vi "err_log.vi"(5 "error IO 2":errorcluster, 6 "time stamp":timestamp) -> (1 "err_table":string[](array[string]))   [LabVIEW 2010]
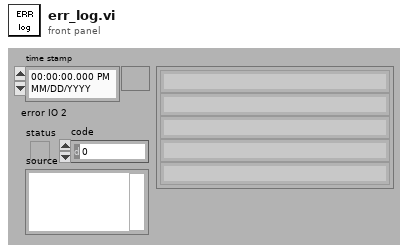
[diagram p1: front panel]
types:
  T1 = enum16{"open", "replace", "create", "open or create", "replace or create", "replace or create with confirmation"}
  T2 = cluster{"status":bool, "code":bool, "source":bool}
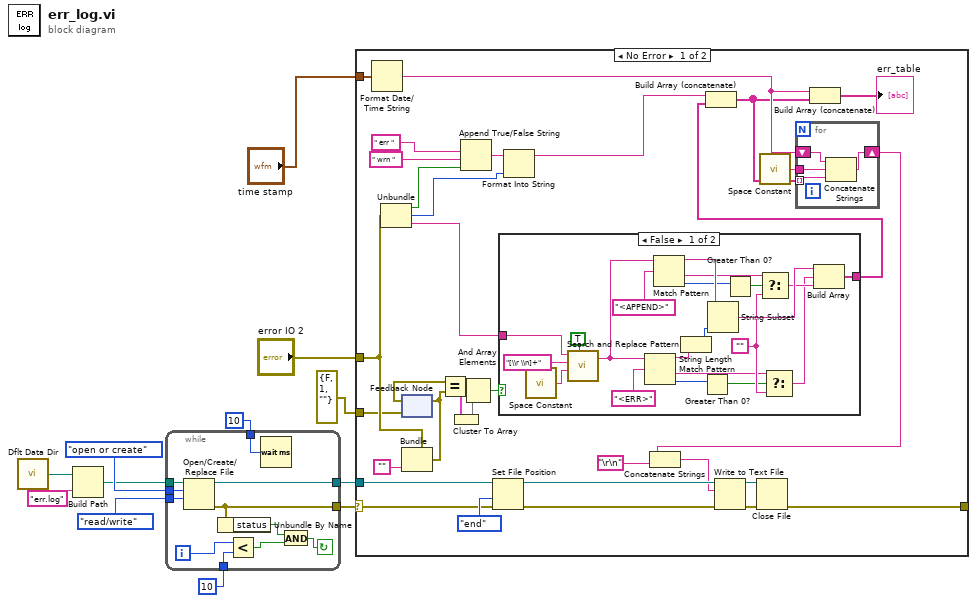
[diagram p0: block diagram]
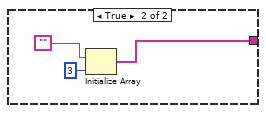
[diagram p2: hidden frame]
diagram:
  n1 = call <vilib>:"Dflt Data Dir.vi"() -> ("App:Default Data Directory"=w9:path)
  n2 = Build Path(base path=w9, name or relative path="err.log") -> (appended path=w10:path)
  n3 = while {
    tunnel: enum16{"read/write", "read-only", "write-only"}."read/write" ("access (0:read/write)") -> [w23]
    tunnel: T1."open or create" ("operation (0:open)") -> [w22]
    tunnel: w10 -> [w21]
    tunnel: [w20] -> w7
    tunnel: 10 ("milliseconds to wait") -> [w18]
    tunnel: u32 10 ("milliseconds to wait") -> [w17]
    tunnel: [w13] -> w4
    i -> [w19]
    stop <- w14 continue-if-true
    n4 = Open/Create/Replace File(file path (use dialog)=w21, operation (0:open)=w22, access (0:read/write)=w23) -> (refnum out=w13:refnum<file>, error out=w20:errorcluster)  [unwired: 3 in, 1 out]
    n5 = Unbundle By Name(w20) -> ("status"=w16:bool)
    n6 = Less?(x=w19, y=w18) -> (x < y?=w15:bool)
    n7 = Wait (ms)(milliseconds to wait=w17) -> ()  [unwired: 1 out]
    n8 = And(x=w16, y=w15) -> (x .and. y?=w14:bool)
  }
  n9 = case shown="No Error" w7 {
    selector: w7 -> [w50 w84]
    tunnel: w4 -> [w49 _]
    tunnel: [w48 w84] -> _
    tunnel: "error IO 2" -> [w38 _]
    tunnel: "time stamp" -> [w37 _]
    tunnel: errorcluster {"status"=FALSE, "code"=1, "source"=""} ("error IO 2") -> [w24 _]
    frame No Error {
      n10 = Format Date/Time String(seconds (now)=w37) -> (date/time string=w30:string)  [unwired: 2 in]
      n11 = Unbundle(w38) -> ("status"=w35:bool, "code"=w34:i32, "source"=w39:string)
      n12 = feedback #1(w24) -> (w42:errorcluster)
      n13 = Bundle(cluster=w38, "source"="") -> (w43:errorcluster)  [unwired: 2 in]
      n14 = feedback-in #1(w43) -> ()
      n15 = Equal?(x=w42, y=w43) -> (x = y?=w41:T2)
      n16 = Cluster To Array(cluster=w41) -> (array=w40:bool[])
      n17 = Append True/False String(1:w35, 2:" wrn ", 3:" err ") -> (0:w45:string)  [unwired: 1 in]
      n18 = And Array Elements(Boolean array=w40) -> (logical AND=w36:bool)
      n19 = Set File Position(refnum=w49, from (0:start)=enum16{"start", "end", "current"}."end", error in=w50) -> (refnum out=w53:refnum<file>, error out=w54:errorcluster)  [unwired: 1 in]
      n20 = case shown="False" w36 {
        tunnel: w39 -> [w76 _]
        tunnel: [w60 w81] -> w31
        frame False {
          w71 = ""
          n21 = call <vilib>:"Space Constant.vi"() -> ("String"=w80:string)
          n22 = call <vilib>:"Search and Replace Pattern.vi"("string"=w76, "regular expression (\"\")"="[\\r \\n]+" ("regular expression (\"\")"), "replace string (\"\")"=w80, "replace all? (F)"=TRUE) -> ("result string"=w77:string)  [unwired: 1 in, 1 out]
          n23 = Match Pattern(string=w77, regular expression="<ERR>" ("search string/char (-)")) -> (before substring=w72:string, after substring=w68:string, offset past match=w67:i32)  [unwired: 1 in, 1 out]
          n24 = Match Pattern(string=w77, regular expression="<APPEND>" ("search string/char (-)")) -> (before substring=w74:string, after substring=w65:string, offset past match=w63:i32)  [unwired: 1 in, 1 out]
          n25 = String Length(string=w72) -> (length=w73:i32)
          n26 = Greater Than 0?(x=w67) -> (x > 0?=w66:bool)
          n27 = String Subset(string=w74, length (rest)=w73) -> (substring=w75:string)  [unwired: 1 in]
          n28 = Greater Than 0?(x=w63) -> (x > 0?=w64:bool)
          n29 = Select(t=w65, s=w64, f=w71) -> (s? t:f=w70:string)
          n30 = Select(t=w68, s=w66, f=w71) -> (s? t:f=w69:string)
          n31 = Build Array(w75, w69, w70) -> (w60:string[])
        }
        frame True {
          n32 = Initialize Array("", 3 ("dimension size")) -> (w81:string[])
        }
      }
      n33 = Format Into String(initial string=w45, w34) -> (resulting string=w32:string)  [unwired: 2 in, 1 out]
      n34 = Build Array (concatenate)(w32, w31) -> (w29:string[])
      n35 = call <vilib>:"Space Constant.vi"() -> ("String"=w33:string)
      n36 = for {
        shift-right: [w59] -> w28
        shift-left: w30 -> [w58]
        tunnel: w29 -> [w57] mode=indexing
        tunnel: w33 -> [w56]
        n37 = Concatenate Strings(w58, w56, w57) -> (w59:string)
      }
      n38 = Concatenate Strings(w28, "\r\n") -> (w26:string)
      n39 = Write to Text File(file (use dialog)=w53, text=w26, error in=w54) -> (refnum out=w51:refnum<file>, error out=w52:errorcluster)  [unwired: 1 in, 1 out]
      n40 = Close File(refnum=w51, error in=w52) -> (error out=w48:errorcluster)  [unwired: 1 out]
      n41 = Build Array (concatenate)(w30, w29) -> (→"err_table":string[])
    }
    frame Error {
    }
  }
